vi "IrDataEventToEventRef.vi"(8 "error in (no error)":errorcluster, 9 "data":T1, 10 "data event in":T7, 11 "TrendPoints Only":bool) -> (0 "error out":errorcluster, 1 "file flow data":T5)   [LabVIEW 2017, in "IrDataEventCreator.lvlib"]
uses:
  <vilib>/addons/InsightCM/Devices/Shared/Ir/IrDataEventCreator/IrDataEventCreator.lvlib
  <vilib>/addons/InsightCM/Devices/Shared/Common/DataEvent/controls/Event.ctl
  <vilib>/addons/InsightCM/MessageBus/Base/controls/DataEvent.ctl
  <vilib>/addons/InsightCM/MessageBus/Base/controls/KeyValuePair.ctl
  <vilib>/addons/InsightCM/Devices/Shared/Common/DataEvent/controls/DataSet.ctl
  <vilib>/addons/InsightCM/MessageBus/Base/controls/DataSetMetadata.ctl
  <vilib>/addons/InsightCM/MessageBus/Base/controls/TrendPoint.ctl
  <vilib>/addons/InsightCM/MessageBus/Base/controls/TrendAlarmUpdate.ctl
  <vilib>/addons/InsightCM/MessageBus/Base/controls/TrendAlarmTransition.ctl
  <vilib>/addons/InsightCM/Devices/Shared/Common/FileFlow/controls/data_eventRef.ctl
  <vilib>/addons/InsightCM/Devices/Shared/Common/DataEvent/controls/EventReference.ctl
  <vilib>/addons/PointValueMap/controls/PointMap.ctl
  <vilib>/addons/InsightCM/Devices/Shared/Common/DataFlow/controls/Data.ctl
  <vilib>/addons/InsightCM/Utilities/DataAccessors/controls/wfmSGL_DVR.ctl
  <vilib>/addons/InsightCM/Devices/Shared/Common/DataFlow/controls/Type.ctl
  <vilib>/addons/PointValueMap/PointValueMap.lvlib
  <vilib>/addons/InsightCM/Devices/Shared/Common/DataEvent/DataEvent.lvlib
  <vilib>/addons/InsightCM/Devices/Shared/Common/FileFlow/FileFlow.lvlib
  <vilib>/addons/InsightCM/Devices/Shared/Common/DataFlow/DataFlow.lvlib
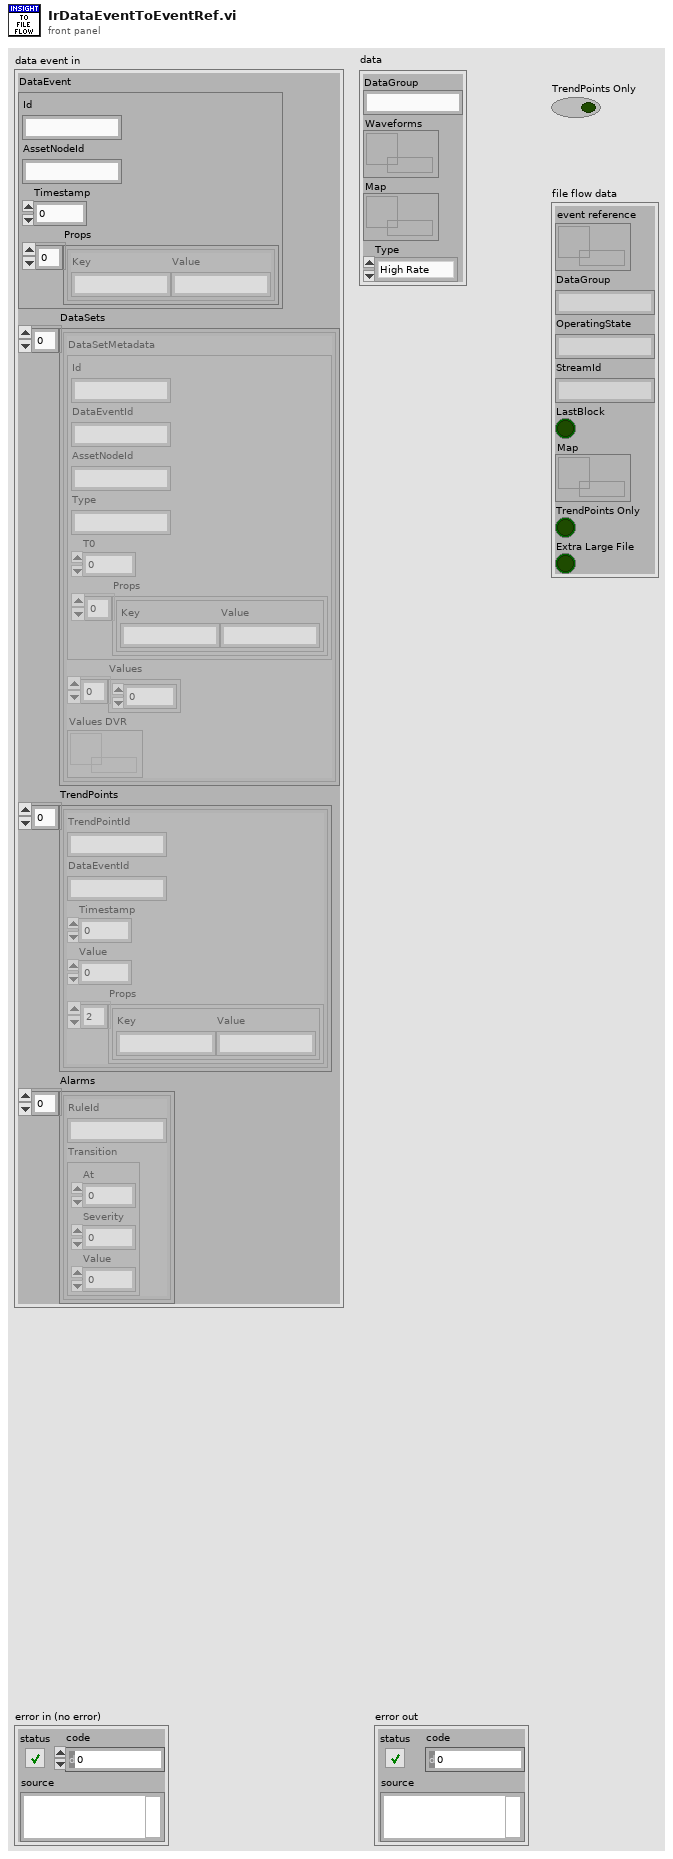
[diagram p1: front panel]
types:
  T1 = typedef "DataFlow.lvlib/Data.ctl" = cluster{"DataGroup":string, "Waveforms":T2, "Map":T3, "Type":T4}
  T2 = typedef "wfmSGL_DVR.ctl" = refnum<data-value>
  T3 = typedef "PointValueMap.lvlib/PointMap.ctl" = refnum<data-value>
  T4 = typedef "DataFlow.lvlib/Type.ctl" = enum16{"High Rate", "Low Rate", "Burst Mode"}
  T5 = typedef "FileFlow.lvlib/data_eventRef.ctl" = cluster{"event reference":T6, "DataGroup":string, "OperatingState":string, "StreamId":string, "LastBlock":bool, "Map":T3, "TrendPoints Only":bool, "Extra Large File":bool}
  T6 = typedef "DataEvent.lvlib/EventReference.ctl" = refnum<data-value>
  T7 = typedef "DataEvent.lvlib/Event.ctl" = cluster{"DataEvent":T8, "DataSets":T10[], "TrendPoints":T12[], "Alarms":T13[]}
  T8 = typedef "DataEvent.ctl" = cluster{"Id":string, "AssetNodeId":string, "Timestamp":i64, "Props":T9[]}
  T9 = typedef "KeyValuePair.ctl" = cluster{"Key":string, "Value":string}
  T10 = typedef "DataEvent.lvlib/DataSet.ctl" = cluster{"DataSetMetadata":T11, "Values":sgl[], "Values DVR":refnum<data-value>}
  T11 = typedef "DataSetMetadata.ctl" = cluster{"Id":string, "DataEventId":string, "AssetNodeId":string, "Type":string, "T0":i64, "Props":T9[]}
  T12 = typedef "TrendPoint.ctl" = cluster{"TrendPointId":string, "DataEventId":string, "Timestamp":i64, "Value":dbl, "Props":T9[]}
  T13 = typedef "TrendAlarmUpdate.ctl" = cluster{"RuleId":string, "Transition":T14}
  T14 = typedef "TrendAlarmTransition.ctl" = cluster{"At":i64, "Severity":i32, "Value":dbl}
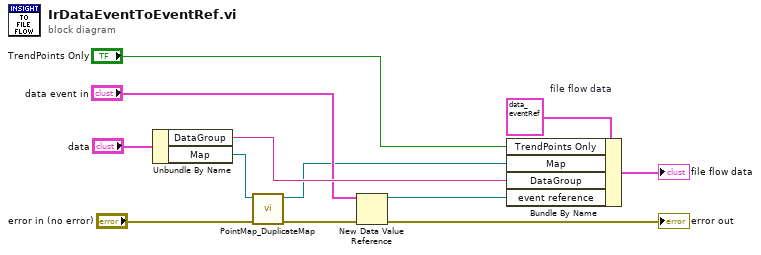
[diagram p0: block diagram]
diagram:
  w9 = T5 {"event reference"=refnum, "DataGroup"="", "OperatingState"="", "StreamId"="", "LastBlock"=FALSE, "Map"=refnum, "TrendPoints Only"=FALSE, "Extra Large File"=FALSE}  # file flow data
  n1 = Unbundle By Name("data") -> ("DataGroup"=w4:string, "Map"=w10:T3)
  n2 = call <vilib>:"PointMap_DuplicateMap.vi"("error in (no error)"="error in (no error)", "map in"=w10) -> ("error out"=w8:errorcluster, "duplicate map"=w2:T3)  [unwired: 8 in]
  n3 = New Data Value Reference(data value="data event in", error in=w8) -> (data value reference=w6:refnum<data-value>, error out=→"error out":errorcluster)
  n4 = Bundle By Name(cluster=w9, "TrendPoints Only"="TrendPoints Only", "Map"=w2, "DataGroup"=w4, "event reference"=w6) -> (→"file flow data":T5)
